vi "get dev number.vi"(8 "error in (no error)":errorcluster, 11 "devs":u16) -> (0 "error out":errorcluster, 2 "function return":bool, 3 "devs out":u16)   [LabVIEW 2015, in "XGL_DPP.lvlib"]
doc: "EXTERN DECLSPEC bool CALL_CONV get_dev_number(unsigned short& devs);"
uses:
  XGL_DPP.lvlib
  D:/Scanning Software_Demokritos_2015_v6/libs/XGL_DPP.dll
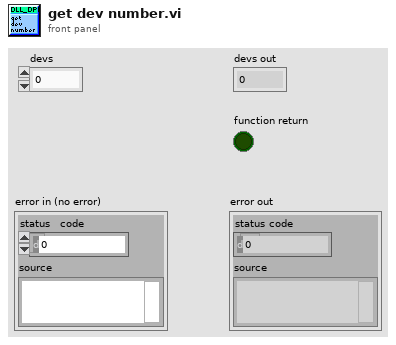
[diagram p1: front panel]
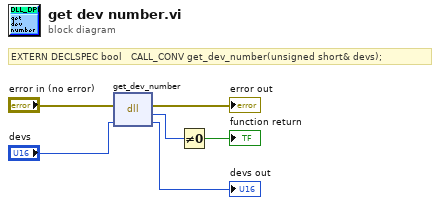
[diagram p0: block diagram]
diagram:
  # "EXTERN DECLSPEC bool   CALL_CONV get_dev_number(unsigned short& devs);"
  n1 = dll-call lib="D:/Scanning Software_Demokritos_2015_v6/libs/XGL_DPP.*" fn="get_dev_number"(error in="error in (no error)", "devs"="devs") -> (error out=→"error out":errorcluster, "return type"=w5:u8, "devs"=→"devs out":u16)  [unwired: 2 in, 1 out]
  n2 = Not Equal To 0?(x=w5) -> (x != 0?=→"function return":bool)
